vi "GetType.vi"(8 "error in (no error)":errorcluster, 11 "Configure BinWidth Msg":refnum<class "Configure BinWidth Msg.lvclass">) -> (0 "error out":errorcluster, 2 "Data Sample":variant, 3 "Configure BinWidth Msg":refnum<class "Configure BinWidth Msg.lvclass">)   [LabVIEW 2016, in "CS++MCS.lvlib" / "Configure BinWidth Msg.lvclass"]
uses:
  Configure BinWidth Msg.lvclass
  Configure BinWidth Msg.lvclass/Configure BinWidth Msg.ctl
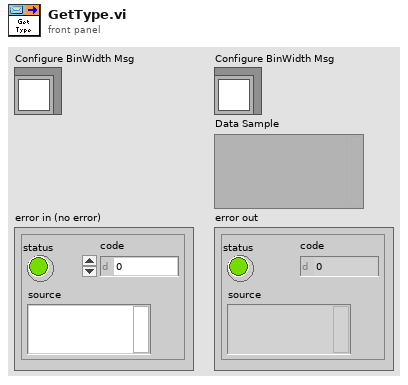
[diagram p1: front panel]
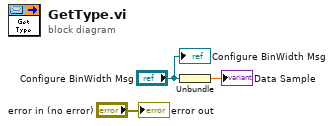
[diagram p0: block diagram]
diagram:
  n1 = Unbundle("Configure BinWidth Msg") -> (→"Data Sample":dbl[unit])
  "error out" <- "error in (no error)"
  "Configure BinWidth Msg" <- "Configure BinWidth Msg"
